vi "GetCCDParameters.vi"(0 "Enable":bool=TRUE, 5 "error in (no error)":errorcluster, 6 "Serial Origin":i32, 7 "Parallel Origin":i32 min=0 step=1, 8 "Serial Length":i32=4096 min=1 step=1, 9 "Parallel Length":i32=4096 caption="Parallel Legnth" min=1 step=1, 10 "Serial Binning":i32=1 min=1 max=4096 step=1, 11 "Parallel Binning":i32=1 min=1 max=4096 step=1) -> (4 "Cancelled?":bool, 14 "CCD Format Parameters":T1, 18 "Set Parameters":bool, 19 "error out":errorcluster)   [LabVIEW 2015]
doc: "Displays a standard dialog box that prompts users to enter information, such as a user name and password.\n--------------------\n\nThis Express VI is configured as follows:\n\nMessage to Display to the User:Please enter CCD Formatting Parameters:\nThe inputs are: \nNumber: Serial Origin\nNumber: Serial Length\nNumber: Serial Binning\nNumber: Parallel Origin\nNumber: Parallel Legnth\nNumber: Parallel Binning"
panel:
  out "Overlap Warning":bool caption="Image Overlap Possible\nIn Serial Direction"
  out "Initial CCD Format Parameters":T1
  in  "y":dbl=1000.0 min=0.0
  in  "x":dbl=1000.0 min=0.0
  in  "Lock ROI Around Object":bool
  in  "Lock To Imaging Region":bool
  in  "Lock To Spectral Region":bool
  in  "Display Spectral Region?":bool
  in  "Display Imaging Circle?":bool
  out "ROI Preview":picture
  out "String":string="Please enter CCD Formatting Parameters:"
  in  "Cancel":bool
  in  "OK2":bool
  in  "OK1":bool
  # "P\na\nr\na\nl\nl\ne\nl"
  # "S   e   r   i   a   l"
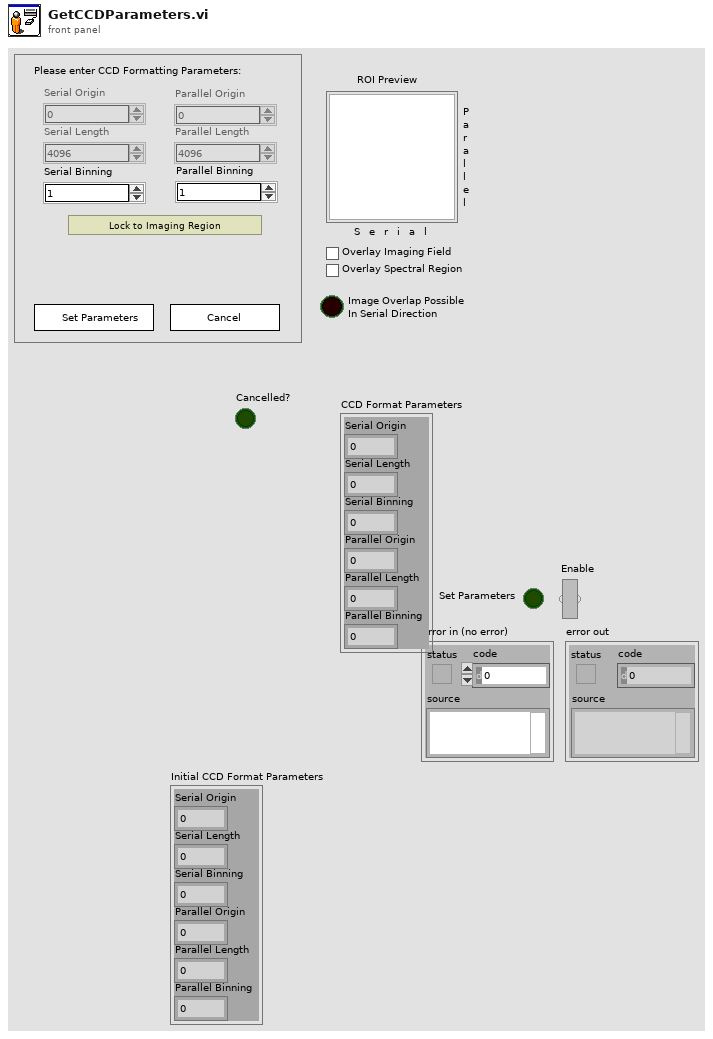
[diagram p1: front panel]
types:
  T1 = cluster{"Serial Origin":i32, "Serial Length":i32, "Serial Binning":i32, "Parallel Origin":i32, "Parallel Length":i32, "Parallel Binning":i32}
  T2 = cluster{"Input Name":string, "Input Data Type":i32}[]
  T3 = cluster{"Width":u16, "Style":enum32{"Solid", "Dash", "Dot", "DashDot", "DashDotDot"}}
  T4 = cluster{"Width":i16, "Style":enum32{"Solid", "Dash", "Dot", "DashDot", "DashDotDot"}}
  T5 = cluster{"Serial Origin":dbl, "Serial Length":i32, "Serial Binning":i32, "Parallel Origin":dbl, "Parallel Length":i32, "Parallel Binning":i32}
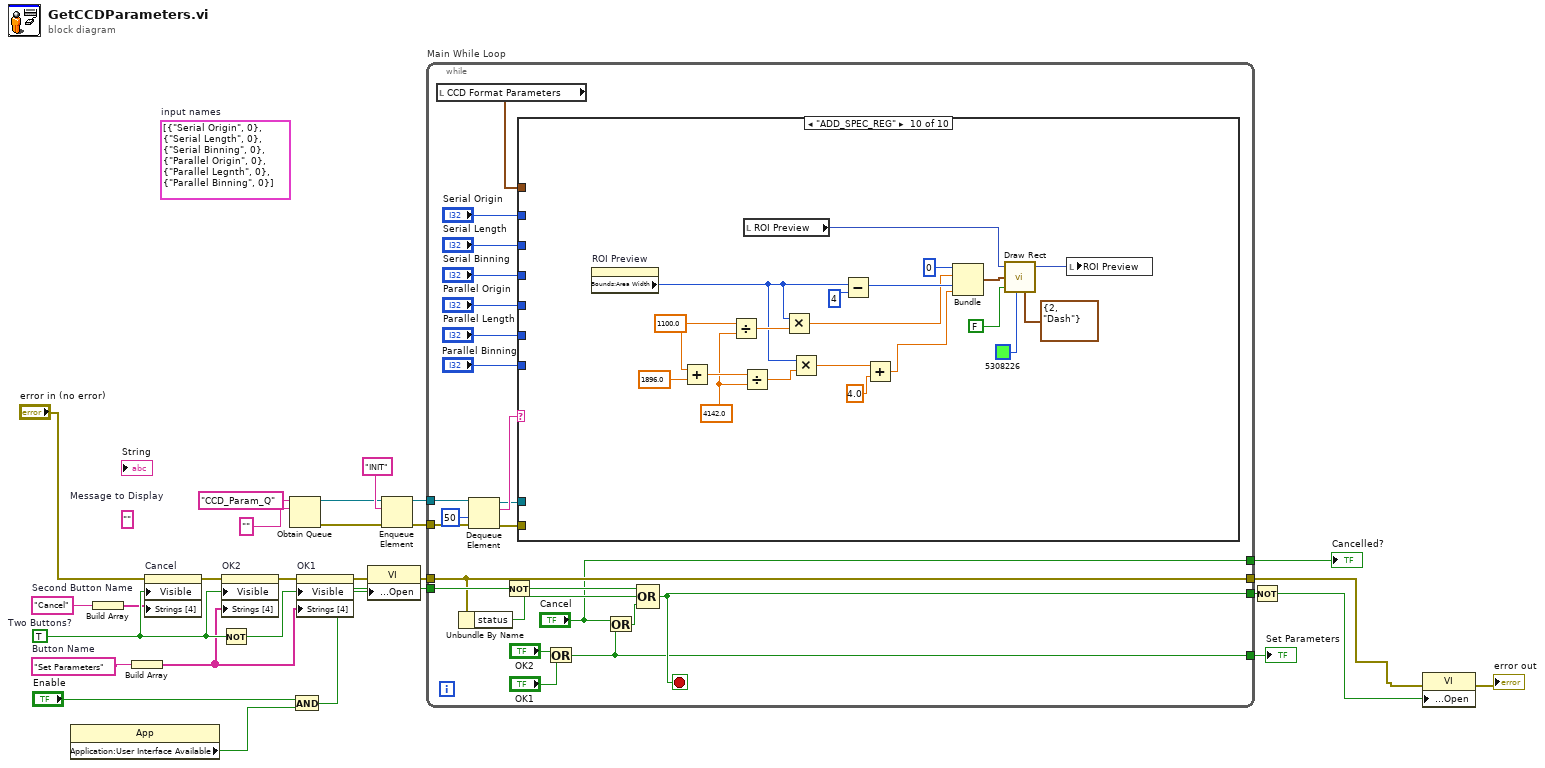
[diagram p0: block diagram]
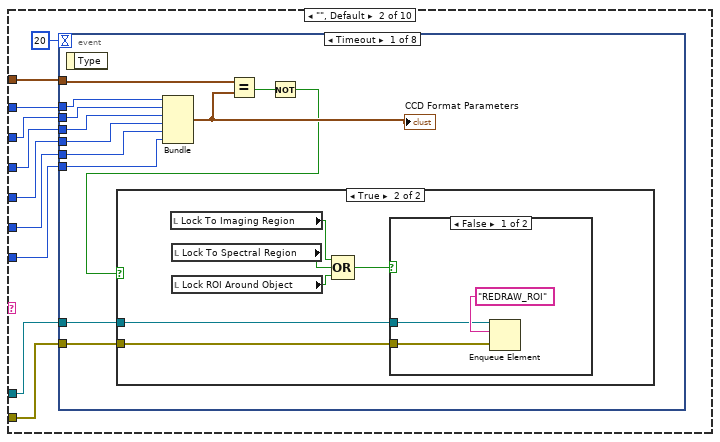
[diagram p3: hidden frame]
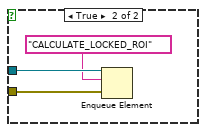
[diagram p5: hidden frame]
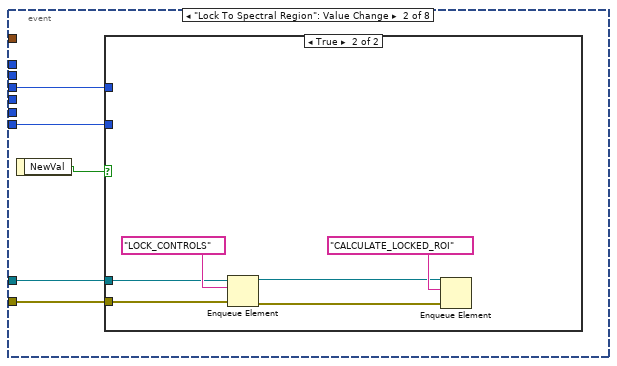
[diagram p6: hidden frame]
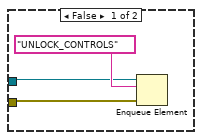
[diagram p7: hidden frame]
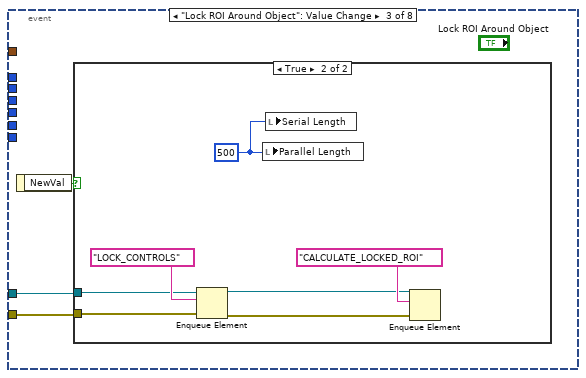
[diagram p8: hidden frame]
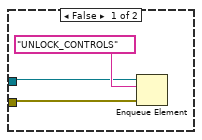
[diagram p9: hidden frame]
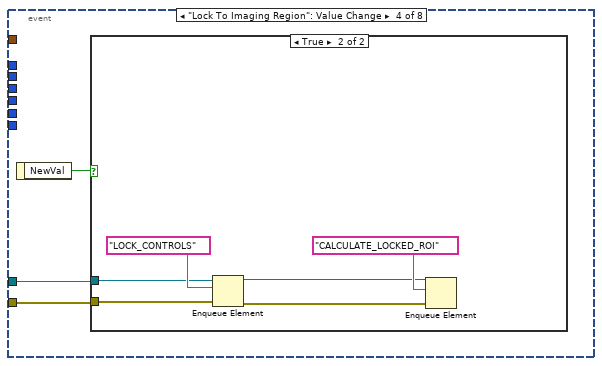
[diagram p10: hidden frame]
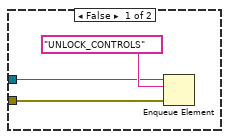
[diagram p11: hidden frame]
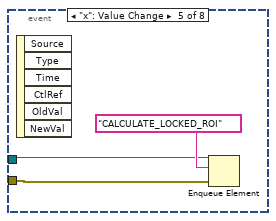
[diagram p12: hidden frame]
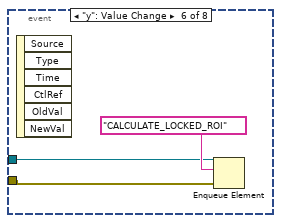
[diagram p13: hidden frame]
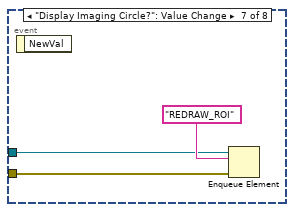
[diagram p14: hidden frame]
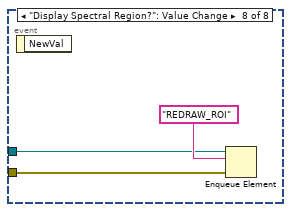
[diagram p15: hidden frame]
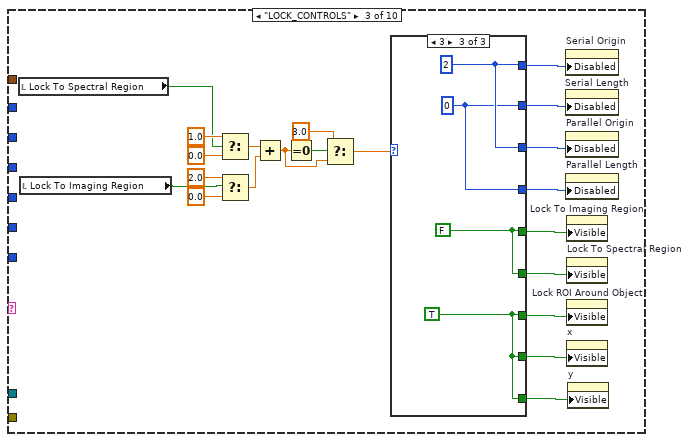
[diagram p16: hidden frame]
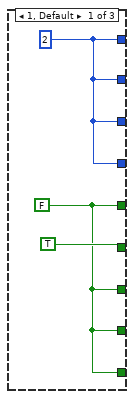
[diagram p17: hidden frame]
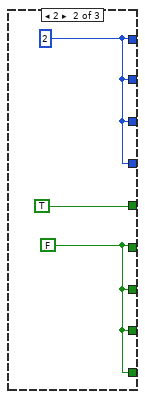
[diagram p18: hidden frame]
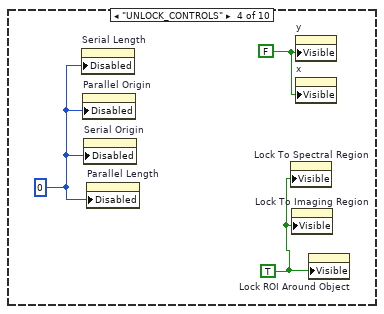
[diagram p19: hidden frame]
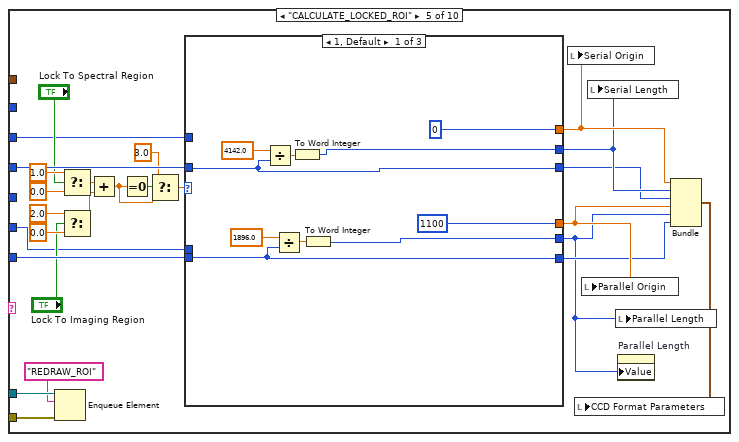
[diagram p20: hidden frame]
diagram:
  (unwired) T2 [{"Input Name"="Serial Origin", "Input Data Type"=0}, {"Input Name"="Serial Length", "Input Data Type"=0}, {"Input Name"="Serial Binning", "Input Data Type"=0}, {"Input Name"="Parallel Origin", "Input Data Type"=0}, {"Input Name"="Parallel Legnth", "Input Data Type"=0}, {"Input Name"="Parallel Binning", "Input Data Type"=0}]  # input names
  w19 = "Cancel"  # Second Button Name
  w17 = "Set Parameters"  # Button Name
  (unwired) ""  # Message to Display
  w27 = TRUE  # Two Buttons?
  n1 = property class="App"() -> ("Application:User Interface Available"=w12:bool)  [unwired: 2 in, 2 out]
  n2 = Build Array(w19) -> (w20:string[])
  n3 = Build Array(w17) -> (w18:string[])
  n4 = property on="Cancel" class="Bool"(error in="error in (no error)", "Visible"=w27, "Strings [4]"=w20) -> (error out=w24:errorcluster)  [unwired: 1 in, 1 out]
  n5 = Not(x=w27) -> (.not. x?=w25:bool)
  n6 = property on="OK2" class="Bool"(error in=w24, "Visible"=w27, "Strings [4]"=w18) -> (error out=w23:errorcluster)  [unwired: 1 in, 1 out]
  n7 = Obtain Queue(name (unnamed)="CCD_Param_Q", element data type="") -> (queue out=w4:refnum<queue>, error out=w3:errorcluster)  [unwired: 3 in, 1 out]
  n8 = And(x="Enable", y=w12) -> (x .and. y?=w13:bool)
  n9 = property on="OK1" class="Bool"(error in=w23, "Visible"=w25, "Strings [4]"=w18) -> (error out=w16:errorcluster)  [unwired: 1 in, 1 out]
  n10 = property class="VI"(error in=w16, "Front Panel Window:Open"=w13) -> (error out=w15:errorcluster)  [unwired: 1 in, 1 out]
  n11 = Enqueue Element(queue=w4, element="INIT", error in (no error)=w3) -> (queue out=w2:refnum<queue>, error out=w1:errorcluster)  [unwired: 1 in, 1 out]
  n12 = while "Main While Loop" {
    tunnel: [w42] -> w26
    tunnel: w13 -> [w48]
    tunnel: [w46] -> w21
    tunnel: w15 -> [w45]
    tunnel: [w45] -> w9
    tunnel: ["Cancel"] -> w11
    tunnel: w2 -> [w40]
    tunnel: w1 -> [w39]
    stop <- w46 stop-if-true
    n13 = local read "CCD Format Parameters"() -> (w28:T1)
    n14 = Unbundle By Name(w45) -> ("status"=w43:bool)
    n15 = Dequeue Element(queue=w40, timeout in ms (-1)=50, error in (no error)=w39) -> (queue out=w35:refnum<queue>, element=w37:string, error out=w36:errorcluster)  [unwired: 1 out]
    n16 = Not(x=w48) -> (.not. x?=w47:bool)
    n17 = case shown="\"ADD_SPEC_REG\"" w37 {
      tunnel: w36 -> [_ w59 _ _ w192 _ _ w260 _ _]
      tunnel: w35 -> [_ w60 _ _ w193 _ _ w261 _ _]
      tunnel: "Serial Origin" -> [_ w58 _ _ _ w243 w259 w273 _ _]
      tunnel: "Serial Length" -> [_ w57 _ _ w172 w246 w258 w278 _ _]
      tunnel: "Serial Binning" -> [_ w56 _ _ w195 w245 w257 w277 _ _]
      tunnel: "Parallel Origin" -> [_ w55 _ _ _ _ w256 w276 _ _]
      tunnel: "Parallel Length" -> [_ w54 _ _ w171 _ w255 w275 _ _]
      tunnel: "Parallel Binning" -> [_ w53 _ _ w194 _ w254 w274 _ _]
      tunnel: w28 -> [_ w52 _ _ _ _ _ _ _ _]
      frame "Draw_Imaging_Circle" {
      }
      frame "", Default {
        n18 = event shown="[0] Timeout" {
          selector: _ -> [_ _ _ _ _ _ _ _]
          dyn-events: _ -> [_ _ _ _ _ _ _ _]
          timeout: 20 -> [_ _ _ _ _ _ _ _]
          tunnel: w58 -> [w72 _ _ _ _ _ _ _]
          tunnel: w56 -> [w71 w88 _ _ _ _ _ _]
          tunnel: w55 -> [w66 _ _ _ _ _ _ _]
          tunnel: w54 -> [w70 _ _ _ _ _ _ _]
          tunnel: w53 -> [w69 w87 _ _ _ _ _ _]
          tunnel: w52 -> [w68 _ _ _ _ _ _ _]
          tunnel: w57 -> [w67 _ _ _ _ _ _ _]
          tunnel: w60 -> [w65 w86 w101 w114 w125 w128 w131 w134]
          tunnel: w59 -> [w64 w85 w100 w113 w124 w127 w130 w133]
          event Timeout {
            n19 = event-data() -> ()  [unwired: 1 in, 1 out]
            n20 = Bundle("Serial Origin"=w72, "Serial Length"=w67, "Serial Binning"=w71, "Parallel Origin"=w66, "Parallel Length"=w70, "Parallel Binning"=w69) -> (w63:T1)  [unwired: 1 in]
            "CCD Format Parameters" <- w63
            n21 = Equal?(x=w68, y=w63) -> (x = y?=w62:bool)
            n22 = Not(x=w62) -> (.not. x?=w61:bool)
            n23 = case shown="True" w61 {
              tunnel: w65 -> [_ w78]
              tunnel: w64 -> [_ w77]
              frame False {
              }
              frame True {
                n24 = local read "Lock To Imaging Region"() -> (w75:bool)
                n25 = local read "Lock To Spectral Region"() -> (w74:bool)
                n26 = local read "Lock ROI Around Object"() -> (w73:bool)
                n27 = Compound Arithmetic op=OR(w75, w74, w73) -> (w76:bool)
                n28 = case shown="False" w76 {
                  tunnel: w78 -> [w80 w84]
                  tunnel: w77 -> [w79 w83]
                  frame False {
                    n29 = Enqueue Element(queue=w80, element="REDRAW_ROI", error in (no error)=w79) -> ()  [unwired: 1 in, 3 out]
                  }
                  frame True {
                    n30 = Enqueue Element(queue=w84, element="CALCULATE_LOCKED_ROI", error in (no error)=w83) -> ()  [unwired: 1 in, 3 out]
                  }
                }
              }
            }
          }
          event "Lock To Spectral Region": Value Change {
            n31 = event-data() -> ("NewVal"=w89:bool)  [unwired: 1 in]
            n32 = case shown="True" w89 {
              tunnel: w88 -> [_ _]
              tunnel: w87 -> [_ _]
              tunnel: w86 -> [w91 w96]
              tunnel: w85 -> [w90 w95]
              frame False {
                n33 = Enqueue Element(queue=w91, element="UNLOCK_CONTROLS", error in (no error)=w90) -> ()  [unwired: 1 in, 3 out]
              }
              frame True {
                n34 = Enqueue Element(queue=w96, element="LOCK_CONTROLS", error in (no error)=w95) -> (queue out=w94:refnum<queue>, error out=w93:errorcluster)  [unwired: 1 in, 1 out]
                n35 = Enqueue Element(queue=w94, element="CALCULATE_LOCKED_ROI", error in (no error)=w93) -> ()  [unwired: 1 in, 3 out]
              }
            }
          }
          event "Lock ROI Around Object": Value Change {
            n36 = event-data() -> ("NewVal"=w99:bool)  [unwired: 1 in]
            n37 = case shown="True" w99 {
              tunnel: w101 -> [w103 w109]
              tunnel: w100 -> [w102 w108]
              frame False {
                n38 = Enqueue Element(queue=w103, element="UNLOCK_CONTROLS", error in (no error)=w102) -> ()  [unwired: 1 in, 3 out]
              }
              frame True {
                w105 = 500 ("Parallel Length")
                n39 = Enqueue Element(queue=w109, element="LOCK_CONTROLS", error in (no error)=w108) -> (queue out=w107:refnum<queue>, error out=w106:errorcluster)  [unwired: 1 in, 1 out]
                n40 = local write "Parallel Length"(w105) -> ()
                n41 = local write "Serial Length"(w105) -> ()
                n42 = Enqueue Element(queue=w107, element="CALCULATE_LOCKED_ROI", error in (no error)=w106) -> ()  [unwired: 1 in, 3 out]
              }
            }
          }
          event "Lock To Imaging Region": Value Change {
            n43 = event-data() -> ("NewVal"=w112:bool)  [unwired: 1 in]
            n44 = case shown="True" w112 {
              tunnel: w114 -> [w116 w121]
              tunnel: w113 -> [w115 w120]
              frame False {
                n45 = Enqueue Element(queue=w116, element="UNLOCK_CONTROLS", error in (no error)=w115) -> ()  [unwired: 1 in, 3 out]
              }
              frame True {
                n46 = Enqueue Element(queue=w121, element="LOCK_CONTROLS", error in (no error)=w120) -> (queue out=w119:refnum<queue>, error out=w118:errorcluster)  [unwired: 1 in, 1 out]
                n47 = Enqueue Element(queue=w119, element="CALCULATE_LOCKED_ROI", error in (no error)=w118) -> ()  [unwired: 1 in, 3 out]
              }
            }
          }
          event "x": Value Change {
            n48 = event-data() -> ()  [unwired: 1 in, 6 out]
            n49 = Enqueue Element(queue=w125, element="CALCULATE_LOCKED_ROI", error in (no error)=w124) -> ()  [unwired: 1 in, 3 out]
          }
          event "y": Value Change {
            n50 = event-data() -> ()  [unwired: 1 in, 6 out]
            n51 = Enqueue Element(queue=w128, element="CALCULATE_LOCKED_ROI", error in (no error)=w127) -> ()  [unwired: 1 in, 3 out]
          }
          event "Display Imaging Circle?": Value Change {
            n52 = event-data() -> ()  [unwired: 1 in, 1 out]
            n53 = Enqueue Element(queue=w131, element="REDRAW_ROI", error in (no error)=w130) -> ()  [unwired: 1 in, 3 out]
          }
          event "Display Spectral Region?": Value Change {
            n54 = event-data() -> ()  [unwired: 1 in, 1 out]
            n55 = Enqueue Element(queue=w134, element="REDRAW_ROI", error in (no error)=w133) -> ()  [unwired: 1 in, 3 out]
          }
        }
      }
      frame "LOCK_CONTROLS" {
        n56 = local read "Lock To Spectral Region"() -> (w150:bool)
        n57 = local read "Lock To Imaging Region"() -> (w149:bool)
        n58 = Select(t=1.0, s=w150, f=0.0) -> (s? t:f=w154:dbl)
        n59 = Select(t=2.0, s=w149, f=0.0) -> (s? t:f=w153:dbl)
        n60 = Add(x=w154, y=w153) -> (x+y=w137:dbl)
        n61 = Equal To 0?(x=w137) -> (x = 0?=w139:bool)
        n62 = Select(t=3.0, s=w139, f=w137) -> (s? t:f=w136:dbl)
        n63 = case shown="3" w136 {
          tunnel: [w159 w162 w166] -> w148
          tunnel: [w159 w162 w165] -> w147
          tunnel: [w159 w162 w166] -> w146
          tunnel: [w159 w162 w165] -> w145
          tunnel: [w157 TRUE w164] -> w144
          tunnel: [TRUE ("Visible") w160 w164] -> w143
          tunnel: [w157 w160 w163] -> w142
          tunnel: [w157 w160 w163] -> w141
          tunnel: [w157 w160 w163] -> w140
          frame 1, Default {
            w157 = FALSE
            w159 = u8 2 ("Disabled")
          }
          frame 2 {
            w160 = FALSE ("Visible")
            w162 = u8 2 ("Disabled")
          }
          frame 3 {
            w165 = u8 0 ("Disabled")
            w163 = TRUE ("Visible")
            w164 = FALSE
            w166 = u8 2 ("Disabled")
          }
        }
        n64 = property on="Serial Origin" class="DigNum (strict)"("Disabled"=w148) -> ()  [unwired: 2 in, 2 out]
        n65 = property on="Serial Length" class="DigNum (strict)"("Disabled"=w147) -> ()  [unwired: 2 in, 2 out]
        n66 = property on="Parallel Origin" class="DigNum (strict)"("Disabled"=w146) -> ()  [unwired: 2 in, 2 out]
        n67 = property on="Parallel Length" class="DigNum (strict)"("Disabled"=w145) -> ()  [unwired: 2 in, 2 out]
        n68 = property on="Lock To Imaging Region" class="Bool (strict)"("Visible"=w144) -> ()  [unwired: 2 in, 2 out]
        n69 = property on="Lock To Spectral Region" class="Bool (strict)"("Visible"=w143) -> ()  [unwired: 2 in, 2 out]
        n70 = property on="Lock ROI Around Object" class="Bool (strict)"("Visible"=w142) -> ()  [unwired: 2 in, 2 out]
        n71 = property on="x" class="DigNum (strict)"("Visible"=w141) -> ()  [unwired: 2 in, 2 out]
        n72 = property on="y" class="DigNum (strict)"("Visible"=w140) -> ()  [unwired: 2 in, 2 out]
      }
      frame "UNLOCK_CONTROLS" {
        w169 = u8 0 ("Disabled")
        w167 = TRUE ("Visible")
        w168 = FALSE ("Visible")
        n73 = property on="Serial Length" class="DigNum (strict)"("Disabled"=w169) -> ()  [unwired: 2 in, 2 out]
        n74 = property on="Parallel Origin" class="DigNum (strict)"("Disabled"=w169) -> ()  [unwired: 2 in, 2 out]
        n75 = property on="Serial Origin" class="DigNum (strict)"("Disabled"=w169) -> ()  [unwired: 2 in, 2 out]
        n76 = property on="Parallel Length" class="DigNum (strict)"("Disabled"=w169) -> ()  [unwired: 2 in, 2 out]
        n77 = property on="Lock To Spectral Region" class="Bool (strict)"("Visible"=w167) -> ()  [unwired: 2 in, 2 out]
        n78 = property on="Lock To Imaging Region" class="Bool (strict)"("Visible"=w167) -> ()  [unwired: 2 in, 2 out]
        n79 = property on="y" class="DigNum (strict)"("Visible"=w168) -> ()  [unwired: 2 in, 2 out]
        n80 = property on="x" class="DigNum (strict)"("Visible"=w168) -> ()  [unwired: 2 in, 2 out]
        n81 = property on="Lock ROI Around Object" class="Bool (strict)"("Visible"=w167) -> ()  [unwired: 2 in, 2 out]
      }
      frame "CALCULATE_LOCKED_ROI" {
        n82 = Enqueue Element(queue=w193, element="REDRAW_ROI", error in (no error)=w192) -> ()  [unwired: 1 in, 3 out]
        n83 = Select(t=1.0, s="Lock To Spectral Region", f=0.0) -> (s? t:f=w182:dbl)
        n84 = Select(t=2.0, s="Lock To Imaging Region", f=0.0) -> (s? t:f=w181:dbl)
        n85 = Add(x=w182, y=w181) -> (x+y=w176:dbl)
        n86 = Equal To 0?(x=w176) -> (x = 0?=w178:bool)
        n87 = Select(t=3.0, s=w178, f=w176) -> (s? t:f=w175:dbl)
        n88 = case shown="1, Default" w175 {
          tunnel: [0 ("Serial Origin") 516 ("Serial Origin") w217] -> w191
          tunnel: [w198 w208 w222] -> w190
          tunnel: [1100 ("Parallel Origin") 500 ("Parallel Origin") w224] -> w188
          tunnel: [w196 w206 w219] -> w185
          tunnel: w195 -> [w201 w211 w221]
          tunnel: w194 -> [w200 w210 w218]
          tunnel: [w201 w211 w221] -> w189
          tunnel: [w200 w210 w218] -> w187
          tunnel: w172 -> [_ _ w222]
          tunnel: w171 -> [_ _ w219]
          frame 1, Default {
            n89 = Divide(x=4142.0, y=w201) -> (x/y=w199:dbl)
            n90 = Divide(x=1896.0, y=w200) -> (x/y=w197:dbl)
            n91 = To Word Integer(number=w199) -> (16bit integer=w198:i16)
            n92 = To Word Integer(number=w197) -> (16bit integer=w196:i16)
          }
          frame 2 {
            n93 = Divide(x=3096.0, y=w211) -> (x/y=w209:dbl)
            n94 = Divide(x=3096.0, y=w210) -> (x/y=w207:dbl)
            n95 = To Word Integer(number=w209) -> (16bit integer=w208:i16)
            n96 = To Word Integer(number=w207) -> (16bit integer=w206:i16)
          }
          frame 3 {
            n97 = local read "Initial CCD Format Parameters"() -> (w238:T1)
            n98 = Multiply(x=w219, y=w218) -> (x*y=w220:i32)
            n99 = Multiply(x=w222, y=w221) -> (x*y=w223:i32)
            n100 = Unbundle(w238) -> ("Serial Origin"=w216:i32, "Serial Binning"=w235:i32, "Parallel Origin"=w231:i32, "Parallel Binning"=w234:i32)  [unwired: 2 out]
            n101 = Divide(x=w220, y=2) -> (x/y=w227:dbl)
            n102 = Multiply(x=w234, y="y") -> (x*y=w232:dbl)
            n103 = Multiply(x=w235, y="x") -> (x*y=w233:dbl)
            n104 = Add(x=w231, y=w232) -> (x+y=w229:dbl)
            n105 = Add(x=w216, y=w233) -> (x+y=w230:dbl)
            n106 = Divide(x=w223, y=2) -> (x/y=w225:dbl)
            n107 = Subtract(x=w229, y=w227) -> (x-y=w224:dbl)
            n108 = Subtract(x=w230, y=w225) -> (x-y=w217:dbl)
          }
        }
        n109 = local write "Serial Origin"(w191) -> ()
        n110 = local write "Parallel Origin"(w188) -> ()
        n111 = local write "Serial Length"(w190) -> ()
        n112 = local write "Parallel Length"(w185) -> ()
        n113 = property on="Parallel Length" class="DigNum (strict)"("Value"=w185) -> ()  [unwired: 2 in, 2 out]
        n114 = Bundle("Serial Origin"=w191, "Serial Length"=w190, "Serial Binning"=w189, "Parallel Origin"=w188, "Parallel Length"=w185, "Parallel Binning"=w187) -> (w186:T5)  [unwired: 1 in]
        n115 = local write "CCD Format Parameters"(w186) -> ()
      }
      frame "CHECK_ROI" {
        n116 = Multiply(x=w246, y=w245) -> (x*y=w244:i32)
        n117 = Add(x=w243, y=w244) -> (x+y=w242:i32)
        n118 = Subtract(x=4096.0, y=w242) -> (x-y=w241:dbl)
        n119 = Greater?(x=w243, y=w241) -> (0:w240:bool)
        n120 = case shown="True" w240 {
          tunnel: [TRUE ("Overlap Warning") FALSE ("Overlap Warning")] -> w239
          frame False {
          }
          frame True {
          }
        }
        "Overlap Warning" <- w239
      }
      frame "INIT" {
        w250 = u8 0 ("Disabled")
        w251 = TRUE ("Visible")
        w252 = FALSE ("Lock ROI Around Object")
        n121 = Bundle("Serial Origin"=w259, "Serial Length"=w258, "Serial Binning"=w257, "Parallel Origin"=w256, "Parallel Length"=w255, "Parallel Binning"=w254) -> (→"Initial CCD Format Parameters":T1)  [unwired: 1 in]
        n122 = property on="Lock To Spectral Region" class="Bool (strict)"("Visible"=w251) -> ()  [unwired: 2 in, 2 out]
        n123 = property on="Lock To Imaging Region" class="Bool (strict)"("Visible"=w251) -> ()  [unwired: 2 in, 2 out]
        n124 = property on="Lock ROI Around Object" class="Bool (strict)"("Visible"=w251) -> ()  [unwired: 2 in, 2 out]
        n125 = local write "Lock To Imaging Region"(w252) -> ()
        n126 = local write "Lock To Spectral Region"(w252) -> ()
        n127 = local write "Lock ROI Around Object"(w252) -> ()
        n128 = property on="y" class="DigNum (strict)"("Visible"=w252) -> ()  [unwired: 2 in, 2 out]
        n129 = property on="Parallel Origin" class="DigNum (strict)"("Disabled"=w250) -> ()  [unwired: 2 in, 2 out]
        n130 = property on="Serial Origin" class="DigNum (strict)"("Disabled"=w250) -> ()  [unwired: 2 in, 2 out]
        n131 = property on="Serial Length" class="DigNum (strict)"("Disabled"=w250) -> ()  [unwired: 2 in, 2 out]
        n132 = property on="Parallel Length" class="DigNum (strict)"("Disabled"=w250) -> ()  [unwired: 2 in, 2 out]
        n133 = property on="x" class="DigNum (strict)"("Visible"=w252) -> ()  [unwired: 2 in, 2 out]
      }
      frame "REDRAW_ROI" {
        w285 = 4096.0 ("y")
        n134 = Enqueue Element(queue=w261, element="CHECK_ROI", error in (no error)=w260) -> (queue out=w263:refnum<queue>, error out=w262:errorcluster)  [unwired: 1 in, 1 out]
        n135 = Multiply(x=w278, y=w277) -> (x*y=w282:i32)
        n136 = Multiply(x=w275, y=w274) -> (x*y=w283:i32)
        n137 = Add(x=w273, y=w282) -> (x+y=w272:i32)
        n138 = Add(x=w276, y=w283) -> (x+y=w286:i32)
        n139 = Subtract(x=w285, y=w286) -> (x-y=w287:dbl)
        n140 = case shown="True" "Display Imaging Circle?" {
          tunnel: w263 -> [w292 w298]
          tunnel: w262 -> [w293 w297]
          tunnel: [w292 w296] -> w268
          tunnel: [w293 w294] -> w267
          frame False {
          }
          frame True {
            n141 = Enqueue Element(queue=w298, element="ADD_IMAGE_REG", error in (no error)=w297) -> (queue out=w296:refnum<queue>, error out=w294:errorcluster)  [unwired: 1 in, 1 out]
          }
        }
        n142 = Subtract(x=w285, y=w276) -> (x-y=w284:dbl)
        n143 = Bundle("Serial Origin"=w273, w287, w272, w284) -> (w280:cluster{"Serial Origin":i32, dbl, i32, dbl})  [unwired: 1 in]
        n144 = property on="ROI Preview" class="Pict"() -> ("Bounds:Area Width"=w271:u32)  [unwired: 2 in, 2 out]
        n145 = Divide(x=w280, y=w285) -> (x/y=w281:cluster{"Serial Origin":dbl, dbl, dbl, dbl})
        n146 = Multiply(x=w271, y=w281) -> (x*y=w288:cluster{"Serial Origin":dbl, dbl, dbl, dbl})
        n147 = call <vilib>:"Draw Rect.vi"("picture"=picture data[5B], "rect"=w288, "fill?(F)"=TRUE) -> ("new picture"=→"ROI Preview":picture)  [unwired: 6 in]
        n148 = case shown="True" "Display Spectral Region?" {
          tunnel: w268 -> [_ w291]
          tunnel: w267 -> [_ w290]
          frame False {
          }
          frame True {
            n149 = Enqueue Element(queue=w291, element="ADD_SPEC_REG", error in (no error)=w290) -> ()  [unwired: 1 in, 3 out]
          }
        }
      }
      frame "ADD_IMAGE_REG" {
        n150 = local read "ROI Preview"() -> (w300:picture)
        n151 = property on="ROI Preview" class="Pict"() -> ("Bounds:Area Width"=w301:u32)  [unwired: 2 in, 2 out]
        n152 = Bundle("Width"=w301, "Width"=w301) -> (w312:cluster{"Width":u32, "Width":u32})  [unwired: 1 in]
        n153 = Divide(x=3096.0, y=2.0) -> (x/y=w306:dbl)
        n154 = Divide(x=w312, y=2 ("Parallel Binning")) -> (x/y=w310:cluster{"Width":dbl, "Width":dbl})
        n155 = Divide(x=w306, y=4096.0) -> (x/y=w305:dbl)
        n156 = Multiply(x=w301, y=w305) -> (x*y=w304:dbl)
        n157 = call <vilib>:"Draw Circle by Radius.vi"("pen"=T3 {"Width"=2, "Style"=enum."Dash"}, "color(black)"=u32 14469632, "pixel center"=w310, "radius"=w304, "picture"=w300) -> ("new picture"=w302:picture)  [unwired: 6 in]
        n158 = local write "ROI Preview"(w302) -> ()
      }
      frame "ADD_SPEC_REG" {
        w324 = 4142.0 ("y")
        w327 = 1100.0 ("x")
        n159 = property on="ROI Preview" class="Pict"() -> ("Bounds:Area Width"=w320:u32)  [unwired: 2 in, 2 out]
        n160 = Add(x=w327, y=1896.0) -> (x+y=w325:dbl)
        n161 = Divide(x=w327, y=w324) -> (x/y=w328:dbl)
        n162 = Divide(x=w325, y=w324) -> (x/y=w323:dbl)
        n163 = local read "ROI Preview"() -> (w321:picture)
        n164 = Multiply(x=w320, y=w328) -> (x*y=w313:dbl)
        n165 = Multiply(x=w320, y=w323) -> (x*y=w315:dbl)
        n166 = Subtract(x=w320, y=u32 4) -> (x-y=w319:u32)
        n167 = Add(x=w315, y=4.0) -> (x+y=w314:dbl)
        n168 = Bundle("Parallel Binning"=0, w313, w319, w314) -> (w332:cluster{"Parallel Binning":i32, dbl, u32, dbl})  [unwired: 1 in]
        n169 = call <vilib>:"Draw Rect.vi"("picture"=w321, "rect"=w332, "fill?(F)"=FALSE, "color(black)"=u32 5308226, "pen"=T4 {"Width"=2, "Style"=enum."Dash"}) -> ("new picture"=w322:picture)  [unwired: 4 in]
        n170 = local write "ROI Preview"(w322) -> ()
      }
    }
    n171 = Or(x="OK2", y="OK1") -> (x .or. y?=w42:bool)
    n172 = Or(x="Cancel", y=w42) -> (x .or. y?=w44:bool)
    n173 = Compound Arithmetic op=OR(w47, w43, w44) -> (w46:bool)
  }
  "Set Parameters" <- w26
  "Cancelled?" <- w11
  n174 = Not(x=w21) -> (.not. x?=w22:bool)
  n175 = property class="VI"(error in=w9, "Front Panel Window:Open"=w22) -> (error out=→"error out":errorcluster)  [unwired: 1 in, 1 out]
